vi "trash_Next Wake Time.vi"() -> ()   [LabVIEW 2021]
uses:
  CIFCore/CIFCoreCommon/CIFCoreCommon.lvlib
  CIFClocks.lvlib
panel:
  out "Sleep Time":i64
  out "Next Target":i64
  in  "Current Time":u64
  in  "Previous target wake":i64
  in  "Offset (us)":i32
  in  "Cycle Rate (s)":dbl
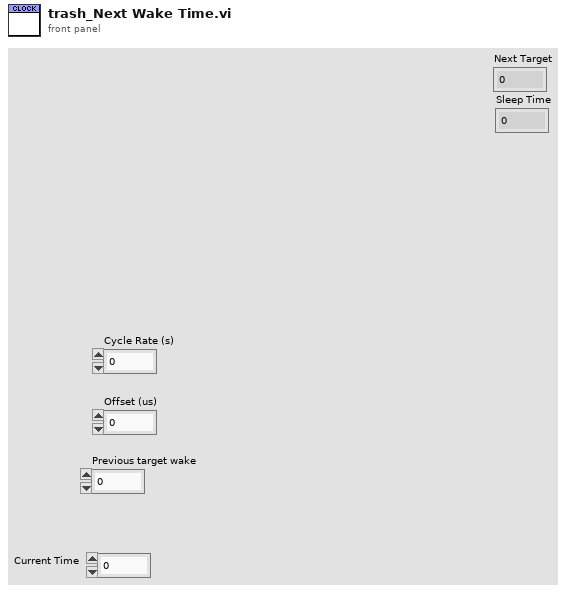
[diagram p1: front panel]
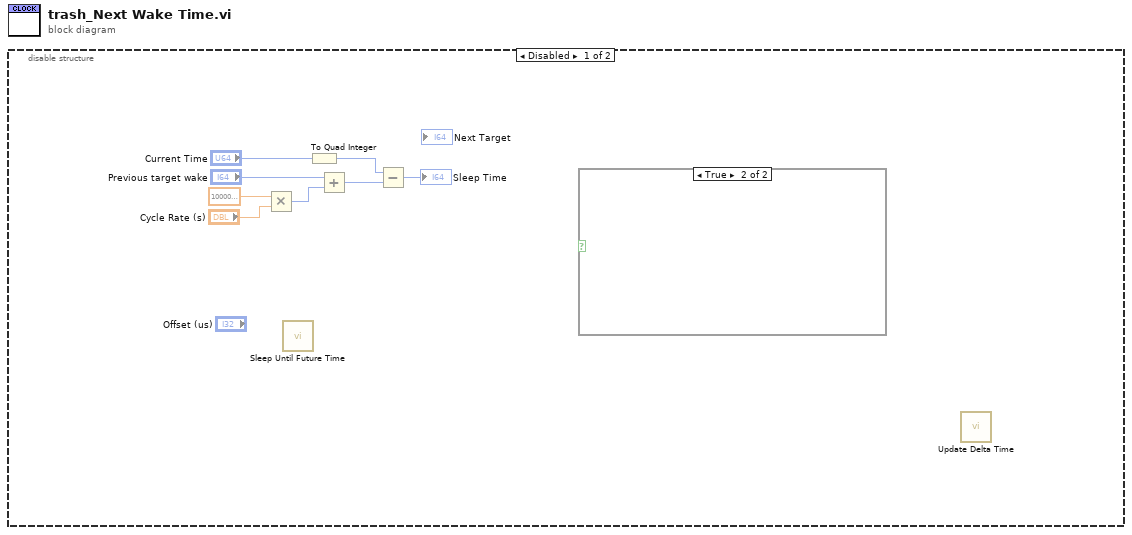
[diagram p0: block diagram]
diagram:
  n1 = disable-structure shown="Disabled" {
    frame Disabled {
      n2 = Multiply(x=1000000000.0, y="Cycle Rate (s)") -> (x*y=w7:i64)
      n3 = call "Sleep Until Future Time.vi"() -> ()  [unwired: 11 in, 1 out]
      n4 = To Quad Integer(1:"Current Time") -> (0:w3:i64)
      n5 = Add(x="Previous target wake", y=w7) -> (x+y=w2:i64)
      n6 = Subtract(x=w3, y=w2) -> (x-y=→"Sleep Time":i64)
      n7 = case shown="True" {
        selector: _ -> [_ _]
        frame False {
        }
        frame True {
        }
      }
      n8 = call "Update Delta Time.vi"() -> ()  [unwired: 10 in, 2 out]
    }
    frame Enabled {
    }
  }
